vi "HEWH GEA2 Set Tank Mode and Temp.vi"(0 "ComPort":refnum<visa-resource-name>="COM1", 5 "Mode":T1=enum."HighDemand", 7 "Set Point":u8=140, 11 "Error In":errorcluster) -> (6 "Mode Read":T1=enum."HighDemand", 8 "SetPoint Read":u8, 15 "Error Out":errorcluster)   [LabVIEW 2014]
uses:
  Utility/GEA2 Commands/HEWH/Type Definitions/HEWH_Mode.ctl
panel:
  out "Current Status Array":string[][](array[string])
  in  "milliseconds to wait":u32=500
  out "Error Out 2":errorcluster
  out "Success":bool
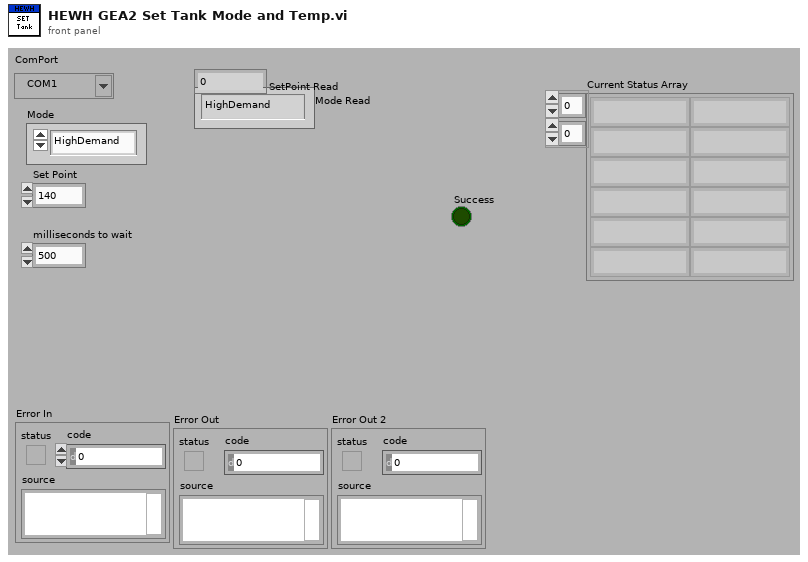
[diagram p1: front panel]
types:
  T1 = typedef "HEWH_Mode.ctl" = enum16{"Hybrid", "Std Electric", "eHeat", "HighDemand", "Vacation"}
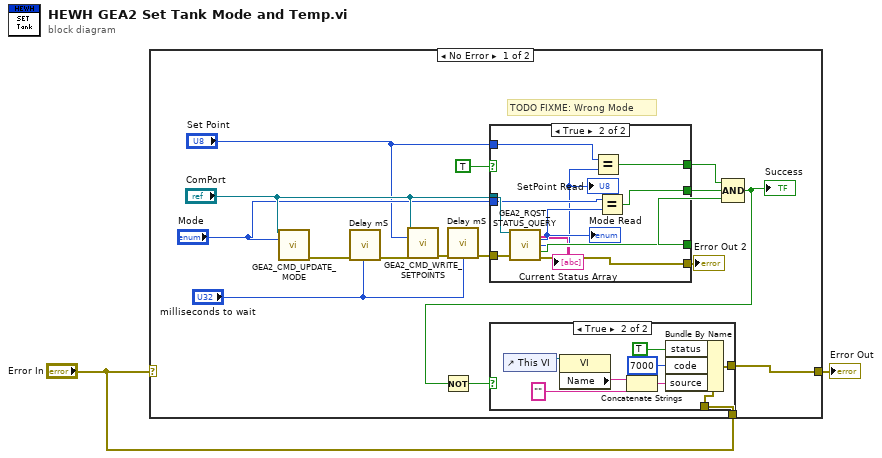
[diagram p0: block diagram]
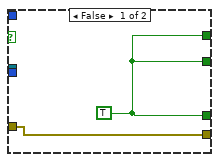
[diagram p2: hidden frame]
diagram:
  n1 = case shown="No Error" "Error In" {
    selector: "Error In" -> [_ w42]
    tunnel: [w19 w42] -> w2
    tunnel: "Error In" -> [w18 _]
    frame No Error {
      # "TODO FIXME: Wrong Mode"
      n2 = call "GEA2_CMD_UPDATE_MODE.vi"("ComPort"="ComPort", "Mode"="Mode") -> ("Error Out"=w9:errorcluster)  [unwired: 11 in, 2 out]
      n3 = call "Delay mS.vi"("Error In"=w9, "milliseconds to wait"="milliseconds to wait") -> ("Error Out"=w6:errorcluster)  [unwired: 13 in]
      n4 = call "GEA2_CMD_WRITE_SETPOINTS.vi"("ComPort"="ComPort", "Set Point"="Set Point", "Error In"=w6) -> ("Error Out"=w8:errorcluster)  [unwired: 11 in, 1 out]
      n5 = call "Delay mS.vi"("Error In"=w8, "milliseconds to wait"="milliseconds to wait") -> ("Error Out"=w7:errorcluster)  [unwired: 13 in]
      n6 = case shown="True" TRUE {
        tunnel: [w21 w32] -> w17
        tunnel: "ComPort" -> [_ w31]
        tunnel: [w20 w30] -> w15
        tunnel: [w20 w29] -> w14
        tunnel: [w20 w28] -> w13
        tunnel: "Mode" -> [_ w26]
        tunnel: "Set Point" -> [_ w24]
        tunnel: w7 -> [w21 w23]
        frame False {
          w20 = TRUE ("CRC Match")
        }
        frame True {
          n7 = call "GEA2_RQST_STATUS_QUERY.vi"("ComPort"=w31, "Error In"=w23) -> ("Current Status Array"=→"Current Status Array":string[][], "Mode"=w27:T1, "Current SetPoint"=w25:u8, "CRC Match"=w30:bool, "Error Out"=w32:errorcluster)  [unwired: 8 in, 1 out]
          "Mode Read" <- w27
          "SetPoint Read" <- w25
          n8 = Equal?(x=w24, y=w25) -> (x = y?=w28:bool)
          n9 = Equal?(x=w26, y=w27) -> (x = y?=w29:bool)
        }
      }
      "Error Out 2" <- w17
      n10 = Compound Arithmetic op=AND(w13, w14, w15) -> (w12:bool)
      "Success" <- w12
      n11 = Not(x=w12) -> (.not. x?=w4:bool)
      n12 = case shown="True" w4 {
        tunnel: [w33 w37] -> w19
        tunnel: w18 -> [w33 w38]
        frame False {
        }
        frame True {
          n13 = control-ref of="This VI"() -> (w41:refnum<vi>)
          n14 = property class="VI"(reference=w41) -> ("Name"=w40:string)  [unwired: 1 in, 2 out]
          n15 = Concatenate Strings(w40, "" ("string")) -> (w35:string)
          n16 = Bundle By Name(cluster=w38, "status"=TRUE, "code"=7000, "source"=w35) -> (w37:errorcluster)
        }
      }
    }
    frame Error {
    }
  }
  "Error Out" <- w2
